vi "setCommandFIFO.vi"(10 "CommandFIFO":refnum<class "IWriteU8FIFO.lvclass">, 11 "RTMockDisplacement in":refnum<class "RTMockDisplacement.lvclass">) -> (3 "RTMockDisplacement out":refnum<class "RTMockDisplacement.lvclass">)   [LabVIEW 2016, in "RTMockDisplacement.lvlib" / "RTMockDisplacement.lvclass"]
uses:
  RTMockDisplacement.lvclass
  Common_RT_FPGA/IWriteU8FIFO/IWriteU8FIFO.lvclass
  RTMockDisplacement.lvclass/RTMockDisplacement.ctl
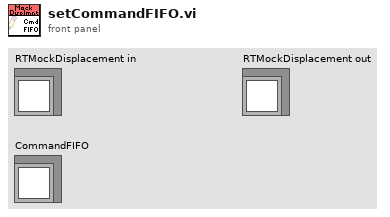
[diagram p1: front panel]
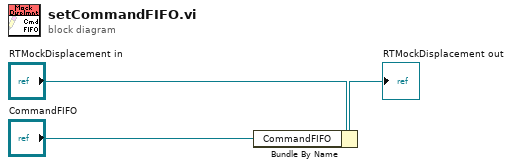
[diagram p0: block diagram]
diagram:
  n1 = Bundle By Name(cluster="RTMockDisplacement in", "CommandFIFO"="CommandFIFO") -> (→"RTMockDisplacement out":refnum<class "RTMockDisplacement.lvclass">)
